vi "Robot hardware Simulator.vi"() -> ()   [LabVIEW 2011]
uses:
  <vilib>/Platform/TimedLoop/XDataNode/timing_clust.ctl
  <vilib>/Platform/TimedLoop/XDataNode/nitl_modes.ctl
  <vilib>/Platform/TimedLoop/XDataNode/wakeup.ctl
  <vilib>/Platform/TimedLoop/XDataNode/XDataNode.xnode
  <vilib>/Platform/TimedLoop/XDataNode/XDNodeRunTimeDep.lvlib
panel:
  out "Wheel Pos/Speed":picture
  in  "Error Correction Speed":dbl
  in  "Engage Simulation":bool
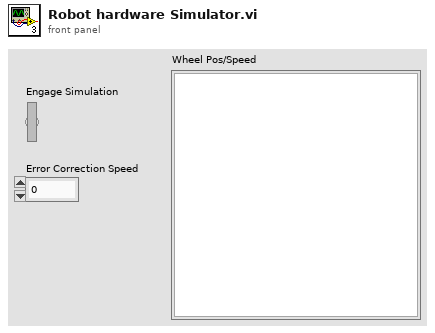
[diagram p1: front panel]
types:
  T1 = typedef "XDNodeRunTimeDep.lvlib/timing_clust.ctl" = cluster{"Expected End [f-1]":u64, "Actual End [f-1]":u64, "Finished Late? [f-1]":bool, "Expected End [i-1]":u64, "Actual End [i-1]":u64, "Finished Late? [i-1]":bool, "Expected Start [i]":u64, "Actual Start [i]":u64, "Expected Start [f]":u64, "Actual Start [f]":u64, "Source Name":string, "Structure Name":string, "Period":i64, "Deadline":i64, "Offset":i64, "Start":i64, "Priority":i32, "Timeout":i32, "Mode":T2, "Wakeup Reason":T3, "Error":errorcluster, "Source Type":string, "Secondary Source Type":string, "Global End Time":u64, "Global Start Time":u64, "Frame Duration":u64, "Iteration Duration":u64, "Assigned CPU":i32, "I/O Scan Engine Mode":u32}
  T2 = typedef "XDNodeRunTimeDep.lvlib/nitl_modes.ctl" = enum32{"No Change", "Process missed periods, maintain original phase", "Discard missed periods, maintain original phase", "Process missed periods, ignore original phase", "Discard missed periods, ignore original phase"}
  T3 = typedef "XDNodeRunTimeDep.lvlib/wakeup.ctl" = enum32{"Normal", "Aborted", "Asynchronous wakeup", "Timing source error", "Timed loop error", "Timeout"}
  T4 = cluster{"Array of Int16[0]":i16, "Array of Int16[1]":i16, "Array of Int16[2]":i16, "Array of Int16[3]":i16, "Array of Int16[4]":i16, "Array of Int16[5]":i16, "Array of Int16[6]":i16, "Array of Int16[7]":i16, "Array of Int16[8]":i16}
  T5 = cluster{"Array of Double[0]":dbl, "Array of Double[1]":dbl, "Array of Double[2]":dbl, "Array of Double[3]":dbl, "Array of Double[4]":dbl, "Array of Double[5]":dbl, "Array of Double[6]":dbl, "Array of Double[7]":dbl, "Array of Double[8]":dbl}
  T6 = cluster{"[0]":dbl, "[1]":dbl, "[2]":dbl, "[3]":dbl, "[4]":dbl, "[5]":dbl, "[6]":dbl, "[7]":dbl, "[8]":dbl}
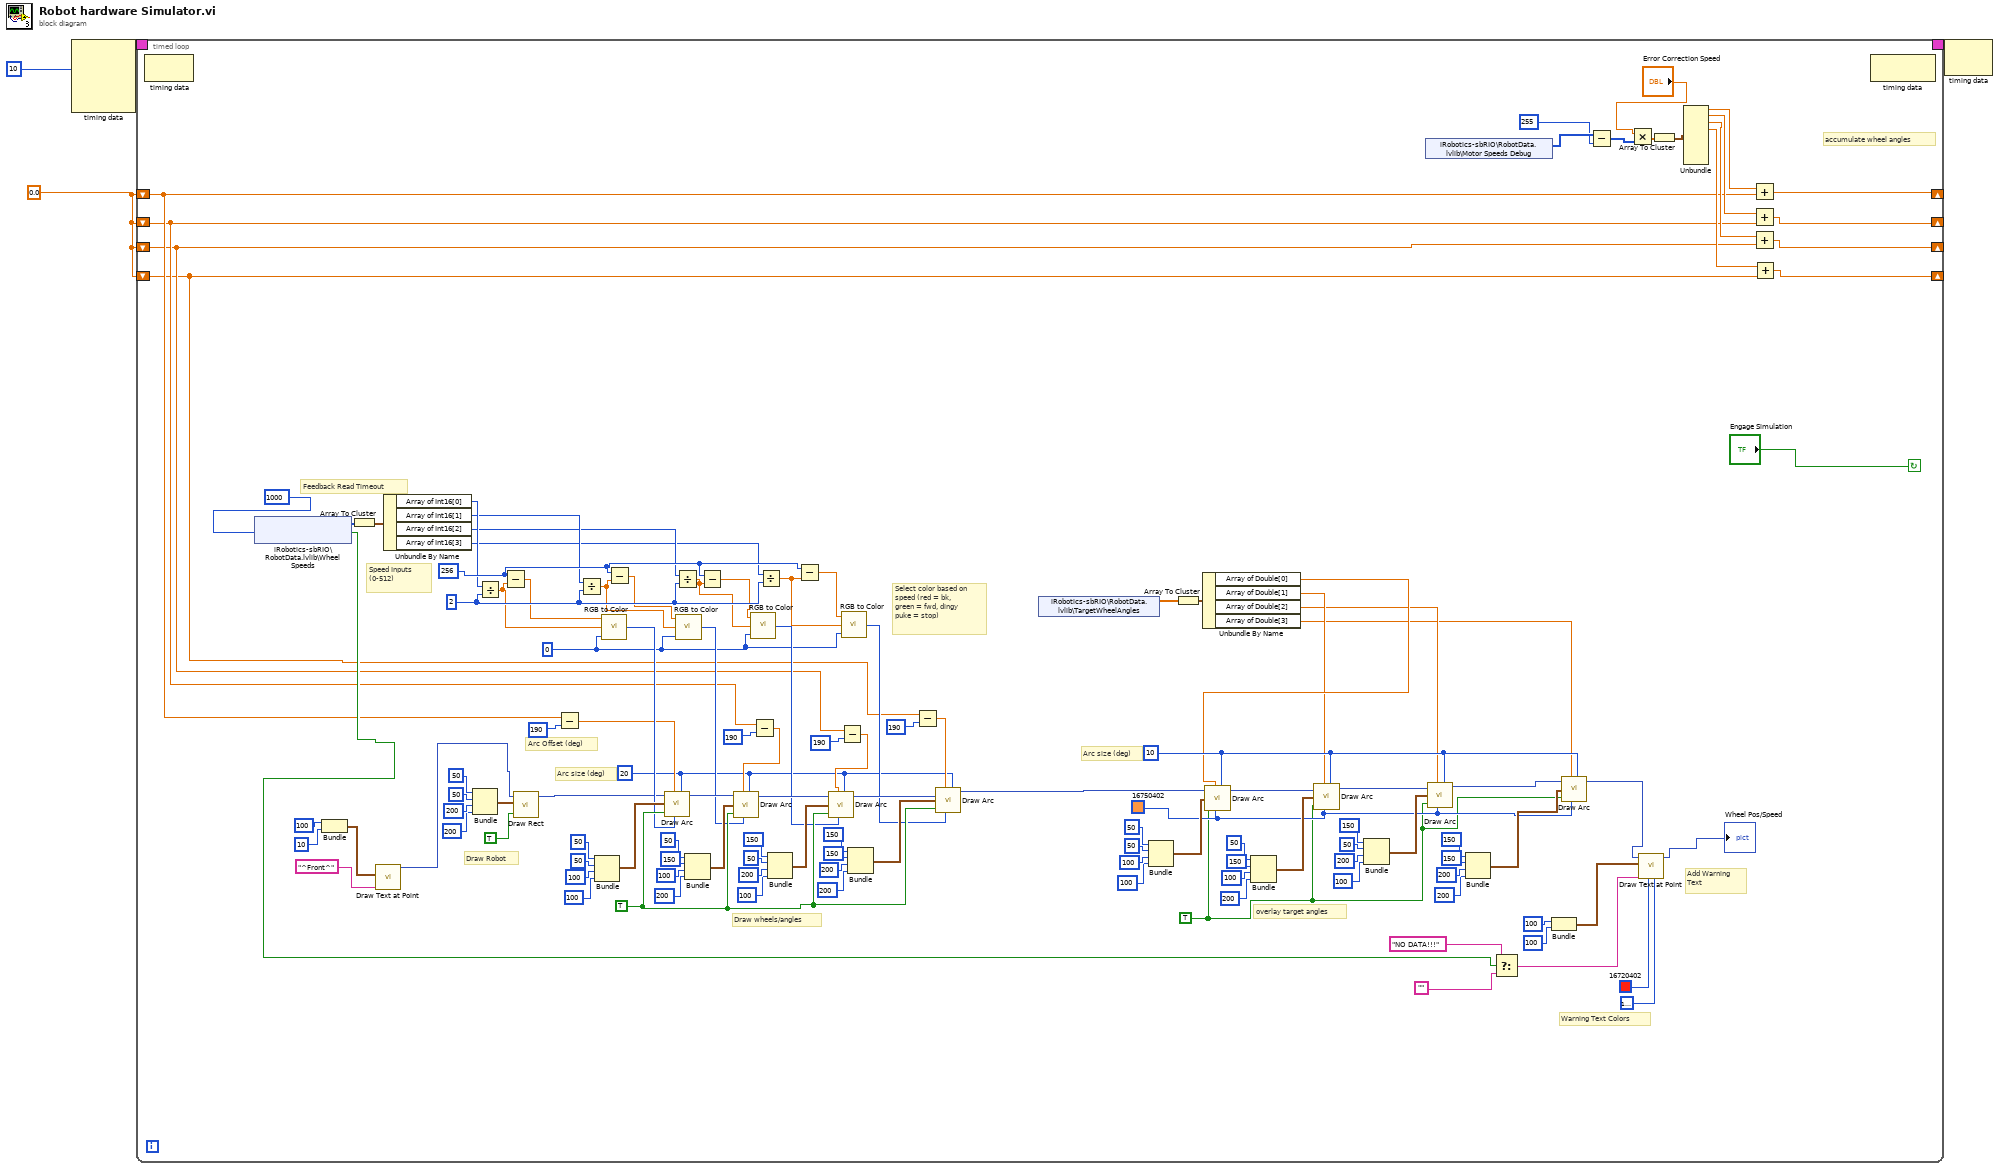
[diagram p0: block diagram]
diagram:
  w1 = 0.0
  n1 = node-c288(10) -> (w4:T1)  [unwired: 3 in]
  n2 = timed-loop {
    timing: w4 -> [_]
    timing-out: [_] -> w3
    shift-right: [w127] -> _
    shift-left: w1 -> [w7]
    shift-right: [w126] -> _
    shift-left: w1 -> [w6]
    shift-right: [w128] -> _
    shift-left: w1 -> [w8]
    shift-right: [w129] -> _
    shift-left: w1 -> [w9]
    stop <- "Engage Simulation" continue-if-true
    w5 = TRUE
    w17 = 10
    w18 = u32 16750402
    w65 = 20
    w67 = 0
    w83 = 2
    w84 = 256
    w96 = TRUE
    # "Arc size (deg)"
    # "overlay target angles"
    # "Add Warning\nText"
    # "Warning Text Colors"
    # "Feedback Read Timeout"
    # "Arc Offset (deg)"
    # "Arc size (deg)"
    # "Speed Inputs (0-512)"
    # "Draw wheels/angles"
    # "Select color based on speed (red = bk, green = fwd, dingy puke = stop)"
    # "Draw Robot"
    # "accumulate wheel angles"
    n3 = node-c288() -> ()  [unwired: 1 in, 1 out]
    n4 = shared-variable "iRobotics-sbRIO\\RobotData.lvlib\\Wheel Speeds"(1000) -> (w59:i16[], w10:bool)  [unwired: 1 in, 1 out]
    n5 = Bundle(100, 10) -> (w60:cluster{i32, i32})  [unwired: 1 in]
    n6 = Array To Cluster(array=w59) -> (cluster=w58:T4)
    n7 = call <vilib>:"Draw Text at Point.vi"("text"="^Front^", "origin"=w60) -> ("new picture"=w64:picture)  [unwired: 8 in, 1 out]
    n8 = Unbundle By Name(w58) -> ("Array of Int16[0]"=w57:i16, "Array of Int16[1]"=w56:i16, "Array of Int16[2]"=w55:i16, "Array of Int16[3]"=w54:i16)
    n9 = Bundle(50, 50, 200, 200) -> (w87:cluster{i32, i32, i32, i32})  [unwired: 1 in]
    n10 = Divide(x=w57, y=w83) -> (x/y=w82:dbl)
    n11 = Subtract(x=w84, y=w82) -> (x-y=w79:dbl)
    n12 = call <vilib>:"Draw Rect.vi"("picture"=w64, "rect"=w87, "fill?(F)"=TRUE) -> ("new picture"=w85:picture)  [unwired: 6 in]
    n13 = Subtract(x=w9, y=190) -> (x-y=w73:dbl)
    n14 = Divide(x=w56, y=w83) -> (x/y=w81:dbl)
    n15 = Bundle(50, 50, 100, 100) -> (w113:cluster{i32, i32, i32, i32})  [unwired: 1 in]
    n16 = call <vilib>:"RGB to Color.vi"("B"=w67, "G"=w82, "R"=w79) -> ("Color"=w95:u32)
    n17 = Subtract(x=w84, y=w81) -> (x-y=w78:dbl)
    n18 = call <vilib>:"Draw Arc.vi"("picture"=w85, "start angle[degrees]"=w73, "rect"=w113, "fill?(F)"=w96, "color(black)"=w95, "arc size[degrees]"=w65) -> ("new picture"=w119:picture)  [unwired: 3 in]
    n19 = Divide(x=w55, y=w83) -> (x/y=w77:dbl)
    n20 = call <vilib>:"RGB to Color.vi"("B"=w67, "G"=w81, "R"=w78) -> ("Color"=w94:u32)
    n21 = Bundle(50, 150, 100, 200) -> (w99:cluster{i32, i32, i32, i32})  [unwired: 1 in]
    n22 = Subtract(x=w84, y=w77) -> (x-y=w76:dbl)
    n23 = call <vilib>:"RGB to Color.vi"("B"=w67, "G"=w77, "R"=w76) -> ("Color"=w93:u32)
    n24 = Subtract(x=w8, y=190) -> (x-y=w69:dbl)
    n25 = call <vilib>:"Draw Arc.vi"("picture"=w119, "start angle[degrees]"=w69, "rect"=w99, "fill?(F)"=w96, "color(black)"=w94, "arc size[degrees]"=w65) -> ("new picture"=w118:picture)  [unwired: 3 in]
    n26 = Divide(x=w54, y=w83) -> (x/y=w80:dbl)
    n27 = Bundle(150, 50, 200, 100) -> (w98:cluster{i32, i32, i32, i32})  [unwired: 1 in]
    n28 = Subtract(x=w84, y=w80) -> (x-y=w75:dbl)
    n29 = Subtract(x=w7, y=190) -> (x-y=w68:dbl)
    n30 = call <vilib>:"Draw Arc.vi"("picture"=w118, "start angle[degrees]"=w68, "rect"=w98, "fill?(F)"=w96, "color(black)"=w93, "arc size[degrees]"=w65) -> ("new picture"=w117:picture)  [unwired: 3 in]
    n31 = call <vilib>:"RGB to Color.vi"("B"=w67, "G"=w80, "R"=w75) -> ("Color"=w92:u32)
    n32 = Bundle(150, 150, 200, 200) -> (w97:cluster{i32, i32, i32, i32})  [unwired: 1 in]
    n33 = Subtract(x=w6, y=190) -> (x-y=w66:dbl)
    n34 = call <vilib>:"Draw Arc.vi"("picture"=w117, "start angle[degrees]"=w66, "rect"=w97, "fill?(F)"=w96, "color(black)"=w92, "arc size[degrees]"=w65) -> ("new picture"=w42:picture)  [unwired: 3 in]
    n35 = shared-variable "iRobotics-sbRIO\\RobotData.lvlib\\TargetWheelAngles"() -> (w15:dbl[])  [unwired: 1 in, 1 out]
    n36 = Bundle(50, 50, 100, 100) -> (w36:cluster{i32, i32, i32, i32})  [unwired: 1 in]
    n37 = Array To Cluster(array=w15) -> (cluster=w16:T5)
    n38 = Unbundle By Name(w16) -> ("Array of Double[0]"=w14:dbl, "Array of Double[1]"=w13:dbl, "Array of Double[2]"=w12:dbl, "Array of Double[3]"=w11:dbl)
    n39 = call <vilib>:"Draw Arc.vi"("picture"=w42, "start angle[degrees]"=w14, "rect"=w36, "fill?(F)"=w5, "color(black)"=w18, "arc size[degrees]"=w17) -> ("new picture"=w41:picture)  [unwired: 3 in]
    n40 = Bundle(50, 150, 100, 200) -> (w30:cluster{i32, i32, i32, i32})  [unwired: 1 in]
    n41 = call <vilib>:"Draw Arc.vi"("picture"=w41, "start angle[degrees]"=w13, "rect"=w30, "fill?(F)"=w5, "color(black)"=w18, "arc size[degrees]"=w17) -> ("new picture"=w24:picture)  [unwired: 3 in]
    n42 = Bundle(150, 50, 200, 100) -> (w25:cluster{i32, i32, i32, i32})  [unwired: 1 in]
    n43 = shared-variable "iRobotics-sbRIO\\RobotData.lvlib\\Motor Speeds Debug"() -> (w133:i16[])  [unwired: 1 in, 1 out]
    n44 = call <vilib>:"Draw Arc.vi"("picture"=w24, "start angle[degrees]"=w12, "rect"=w25, "fill?(F)"=w5, "color(black)"=w18, "arc size[degrees]"=w17) -> ("new picture"=w40:picture)  [unwired: 3 in]
    n45 = Bundle(150, 150, 200, 200) -> (w19:cluster{i32, i32, i32, i32})  [unwired: 1 in]
    n46 = Select(t="NO DATA!!!", s=w10, f="") -> (s? t:f=w46:string)
    n47 = Bundle(100, 100) -> (w50:cluster{i32, i32})  [unwired: 1 in]
    n48 = call <vilib>:"Draw Arc.vi"("picture"=w40, "start angle[degrees]"=w11, "rect"=w19, "fill?(F)"=w5, "color(black)"=w18, "arc size[degrees]"=w17) -> ("new picture"=w43:picture)  [unwired: 3 in]
    n49 = Subtract(x=w133, y=255) -> (x-y=w131:i32[])
    n50 = Multiply(x="Error Correction Speed", y=w131) -> (x*y=w125:dbl[])
    n51 = call <vilib>:"Draw Text at Point.vi"("BG color(transparent)"=u32 16777216, "text color(black)"=u32 16720402, "text"=w46, "origin"=w50, "picture"=w43) -> ("new picture"=→"Wheel Pos/Speed":picture)  [unwired: 5 in, 1 out]
    n52 = Array To Cluster(array=w125) -> (cluster=w130:T6)
    n53 = Unbundle(w130) -> ("[0]"=w123:dbl, "[1]"=w122:dbl, "[2]"=w121:dbl, "[3]"=w120:dbl)  [unwired: 5 out]
    n54 = Add(x=w123, y=w9) -> (x+y=w129:dbl)
    n55 = Add(x=w122, y=w8) -> (x+y=w128:dbl)
    n56 = Add(x=w121, y=w7) -> (x+y=w127:dbl)
    n57 = Add(x=w120, y=w6) -> (x+y=w126:dbl)
    n58 = node-c288() -> ()  [unwired: 1 in, 1 out]
  }
  n59 = node-c288(w3) -> ()  [unwired: 1 out]
